vi "One Dynamic Input One Dynamic Output.vi"(8 "error in (no error)":errorcluster, 11 "Class Gamma in":refnum<class "Class Gamma.lvclass">) -> (0 "error out":errorcluster, 3 "Class Gamma out":refnum<class "Class Gamma.lvclass">)   [LabVIEW 2023, in "Class Gamma.lvclass"]
doc: "This VI overrides the VI of the same name in Class Alpha."
uses:
  Class Gamma.lvclass
  Class Gamma.lvclass/Class Gamma.ctl
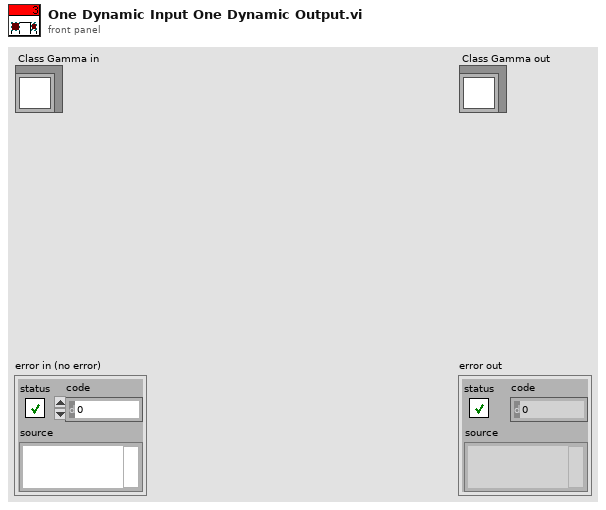
[diagram p1: front panel]
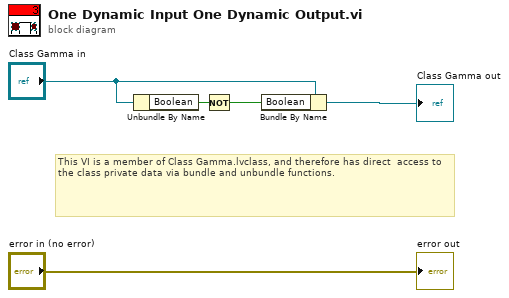
[diagram p0: block diagram]
diagram:
  # "This VI is a member of Class Gamma.lvclass, and therefore has direct  access to the class private data via bundle and unbundle functions."
  n1 = Unbundle By Name("Class Gamma in") -> ("Boolean"=w4:bool)
  n2 = Not(x=w4) -> (.not. x?=w2:bool)
  n3 = Bundle By Name(cluster="Class Gamma in", "Boolean"=w2) -> (→"Class Gamma out":refnum<class "Class Gamma.lvclass">)
  "error out" <- "error in (no error)"
